vi "ziGetVoltageCalcVal.vi"(8 "Imp50":bool, 9 "VGain":i32, 10 "Voltage (Vrms)":cdb format="%#_6p", 11 "Mode":enum16{"From Sig Out", "Signal Input", "HF2CA"}(ring)) -> (2 "Vz (Vrms)":cdb format="%#_6p")   [LabVIEW 2009, in "Zurich Instruments LabOne.lvlib"]
uses:
  <instrlib>/Zurich Instruments LabOne/Zurich Instruments LabOne.lvlib
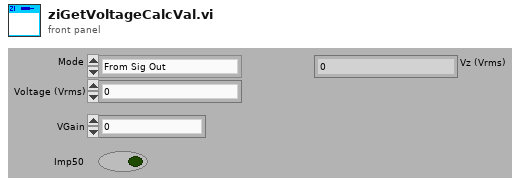
[diagram p1: front panel]
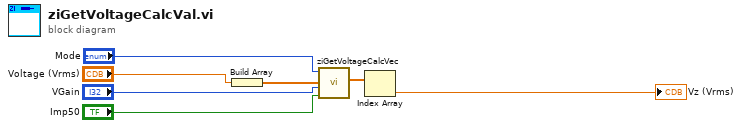
[diagram p0: block diagram]
diagram:
  n1 = Build Array("Voltage (Vrms)") -> (w6:cdb[])
  n2 = call <instrlib>:"ziGetVoltageCalcVec.vi"("Imp50 (F)"="Imp50", "VGain"="VGain", "DemodVoltage (Vrms)"=w6, "Mode"="Mode") -> ("Vz (Vrms)"=w1:cdb[])  [unwired: 7 in]
  n3 = Index Array(array=w1) -> (element=→"Vz (Vrms)":cdb)  [unwired: 1 in]
